vi "State_Machine.vi"(8 "error in (no error)":errorcluster caption="entrée d'erreur (pas d'erreur)", 11 "Wait_CloseFixture en entrée":refnum<class "Hide_Operator_Information.lvclass">) -> (0 "error out":errorcluster caption="sortie d'erreur", 2 "Json_String":string, 3 "Wait_CloseFixture en sortie":refnum<class "Hide_Operator_Information.lvclass">)   [LabVIEW 2020, in "Library Test.lvlib" / "Hide_Operator_Information.lvclass"]
uses:
  Hide_Operator_Information.lvclass
  Popup/Class Popup Operator_Validation/Class Popup Operator_Information/Class Popup Operator_Information.lvclass
  C:/Users/ngarcin/OneDrive - Altyor/Standard TB/Suite TB45/Class/Popup/Class Popup (Main)/Class Popup (Main).lvclass
  Commun VI/TypeDef/Variable Printable.ctl
  JSON API/JSON Value/Set from JSON string.vi
  JSON API/JSON Value/JSON Value.lvclass
  Commun VI/Library Commun.lvlib
  JSON API/Get Polymorphic/JSON GetSet.lvlib
  JSON API/Variant JSON/Variant JSON.lvlib
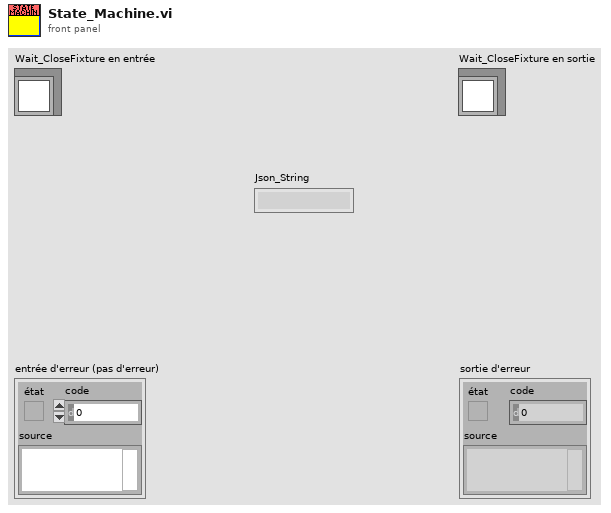
[diagram p1: front panel]
types:
  T1 = enum16{"Get Variable", "Get All Variables", "Set Variable", "Delete Variable", "Delete All Variable"}
  T2 = typedef "Variable Printable.ctl" = string
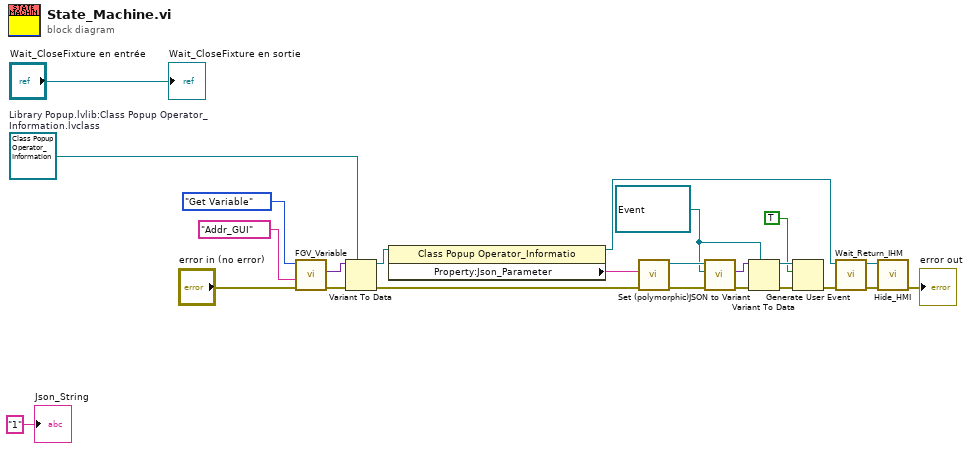
[diagram p0: block diagram]
diagram:
  w8 = refnum<user-event> refnum ("événement utilisateur de sortie")
  w12 = refnum<class "Class Popup Operator_Information.lvclass"> refnum  # Library Popup.lvlib:Class Popup Operator_Information.lvclass
  n1 = call "FGV_Variable.vi"("error in (no error)"="error in (no error)", "Variable"=T2 "Addr_GUI", "Function"=T1."Get Variable") -> ("error out"=w13:errorcluster, "Data Out"=w11:variant)  [unwired: 6 in, 1 out]
  n2 = Variant To Data(error in=w13, type=w12, Variant=w11) -> (data=w10:refnum<class "Class Popup Operator_Information.lvclass">, error out=w7:errorcluster)
  n3 = property class="Class Popup Operator_Informatio"(reference=w10) -> (reference out=w1:refnum<class "Class Popup Operator_Information.lvclass">, "Property:Json_Parameter"=w14:string)  [unwired: 1 in, 1 out]
  n4 = call-poly "Set (polymorphic).vi"("error in (no error)"=w7, "JSON stream"=w14) -> ("error out"=w16:errorcluster, "JSON Value out"=w18:refnum<class "JSON Value.lvclass">)  [unwired: 7 in, 1 out]
  n5 = call "JSON to Variant.vi"("error in (no error)"=w16, "Variant (Data Type)"=w8, "JSON Value"=w18) -> ("error out"=w17:errorcluster, "Variant out"=w15:variant)  [unwired: 7 in]
  n6 = Variant To Data(error in=w17, type=w8, Variant=w15) -> (data=w5:refnum<user-event>, error out=w6:errorcluster)
  n7 = Generate User Event(user event=w5, event data cluster=TRUE ("données d'événement"), error in=w6) -> (error out=w3:errorcluster)  [unwired: 1 in, 1 out]
  n8 = call-dynamic "Wait_Return_IHM.vi"("error in (no error)"=w3, "Class Popup (Default) en entrée"=w1) -> ("error out"=w21:errorcluster, "Class Popup (Default) en sortie"=w22:refnum<class "Class Popup Operator_Information.lvclass">)  [unwired: 8 in]
  n9 = call-dynamic "Hide_HMI.vi"("error in (no error)"=w21, "Class Popup (Default) en entrée"=w22) -> ("error out"=→"error out":errorcluster)  [unwired: 8 in, 1 out]
  "Wait_CloseFixture en sortie" <- "Wait_CloseFixture en entrée"
  "Json_String" <- "1"
